vi "Send to Peer.vi"(7 "timeout ms (5000)":i32=5000, 8 "error in (no error)":errorcluster, 9 "Data Format (Text)":T1, 10 "Data":string, 11 "WebSocket Connection in":refnum<class "WebSocket Connection.lvclass">) -> (0 "error out":errorcluster, 3 "WebSocket Connection out":refnum<class "WebSocket Connection.lvclass">)   [LabVIEW 2017, in "WebSocket Actors.lvlib" / "WebSocket Connection.lvclass"]
doc: "This method sends data to the connected peers in either text or binary format"
uses:
  WebSocket Connection.lvclass
  Websockets/Data Format.ctl
  WebSocket Connection.lvclass/WebSocket Connection.ctl
  <vilib>/GPower/Error/Library/SplitAppended.vi
  <vilib>/GPower/Error/Library/AppendErrors.vi
  <vilib>/GPower/Error/Library/Append/AppendMulti.vi
  <vilib>/GPower/Error/Library/SubVIs/ExplanationToError.vi
  <vilib>/dlg_ctls.llb/Space Constant.vi
  <vilib>/Utility/error.llb/Trim Whitespace.vi
  <vilib>/Utility/error.llb/Error Code Database.vi
  <vilib>/GPower/Error/Library/Append/AppendSingle.vi
  Websockets/LV WebSockets.lvlib
  <vilib>/GPower/Error/GPError.lvlib
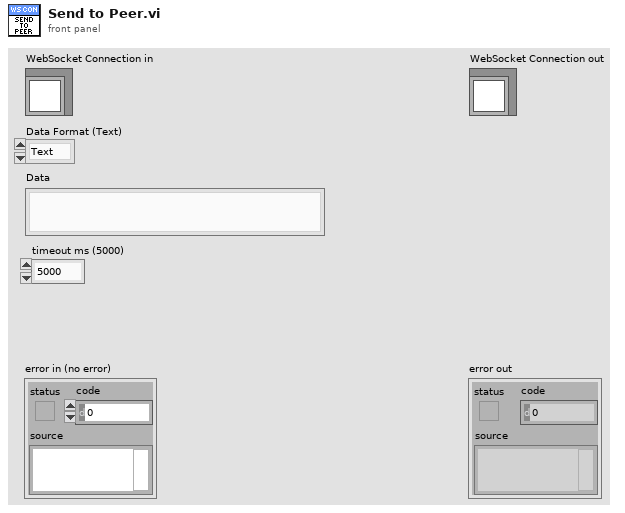
[diagram p1: front panel]
types:
  T1 = typedef "LV WebSockets.lvlib/Data Format.ctl" = enum16{"Text", "Binary"}
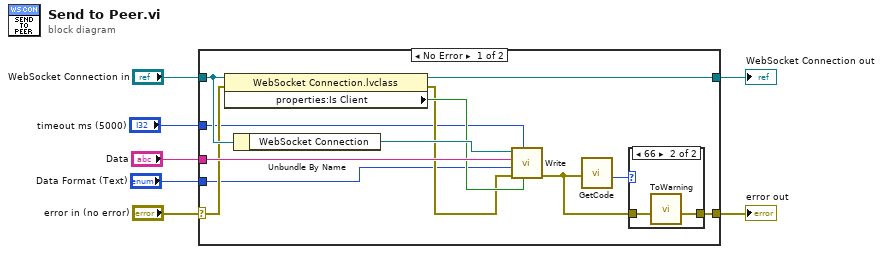
[diagram p0: block diagram]
diagram:
  n1 = case shown="No Error" "error in (no error)" {
    selector: "error in (no error)" -> [w14 w24]
    tunnel: [w9 w24] -> w6
    tunnel: [w16 w23] -> w4
    tunnel: "WebSocket Connection in" -> [w19 w23]
    tunnel: "Data" -> [w17 _]
    tunnel: "timeout ms (5000)" -> [w12 _]
    tunnel: "Data Format (Text)" -> [w11 _]
    frame No Error {
      n2 = property class="WebSocket Connection.lvclass"(reference=w19, error in=w14) -> (reference out=w16:refnum<class "WebSocket Connection.lvclass">, error out=w13:errorcluster, "properties:Is Client"=w15:bool)
      n3 = Unbundle By Name(w19) -> ("WebSocket Connection"=w18:refnum<k5>)
      n4 = call "Write.vi"("Mask payload?"=w15, "timeout ms (5000)"=w12, "error in (no error)"=w13, "Data Format (Text)"=w11, "Data"=w17, "WebSocket Connection in"=w18) -> ("error out"=w8:errorcluster)  [unwired: 4 in, 1 out]
      n5 = call <vilib>:"GetCode.vi"("Error in"=w8) -> ("Code"=w10:i32)  [unwired: 10 in]
      n6 = case shown="66" w10 {
        tunnel: [w20 w21] -> w9
        tunnel: w8 -> [w20 w22]
        frame Default {
        }
        frame 66 {
          n7 = call <vilib>:"ToWarning.vi"("Error in"=w22) -> ("Warning out"=w21:errorcluster)  [unwired: 10 in]
        }
      }
    }
    frame Error {
    }
  }
  "error out" <- w6
  "WebSocket Connection out" <- w4
